vi "Add_DB_info_to_Raw_Data.vi"() -> (0 "Filename":path, 1 "Channel names":string[](array[string]), 2 "Valid File?":bool, 3 "Ch Values":string[][](table))   [LabVIEW 2010]
panel:
  in  "Comment to add":string=" Manually removed"
  in  "Scale Channels":bool
  in  "Scaling Factor":dbl[](array[numeric]) format="%.4f"
  in  "Channel Numbers":i32[](array[numeric])
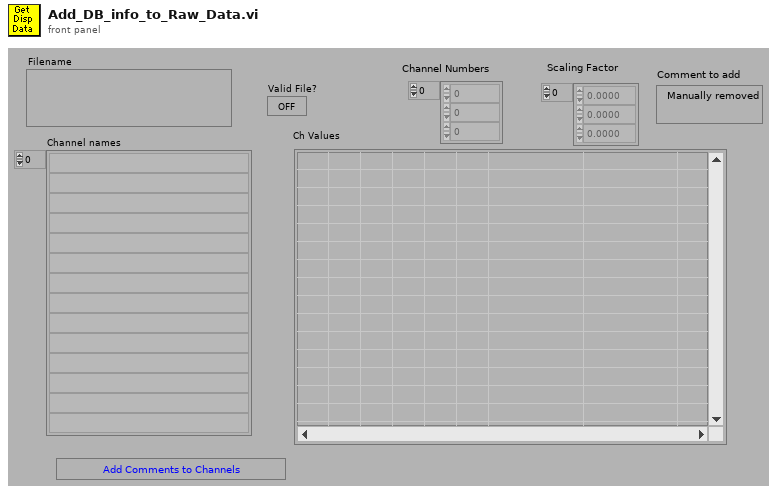
[diagram p1: front panel]
types:
  T1 = enum32{"existing file", "new file", "new or existing file", "existing dir", "new dir", "new or existing dir", "existing file (use LLBs)", "new file (use LLBs)", "new or existing file (use LLBs)", "new or existing file or directory (use LLBs)"}
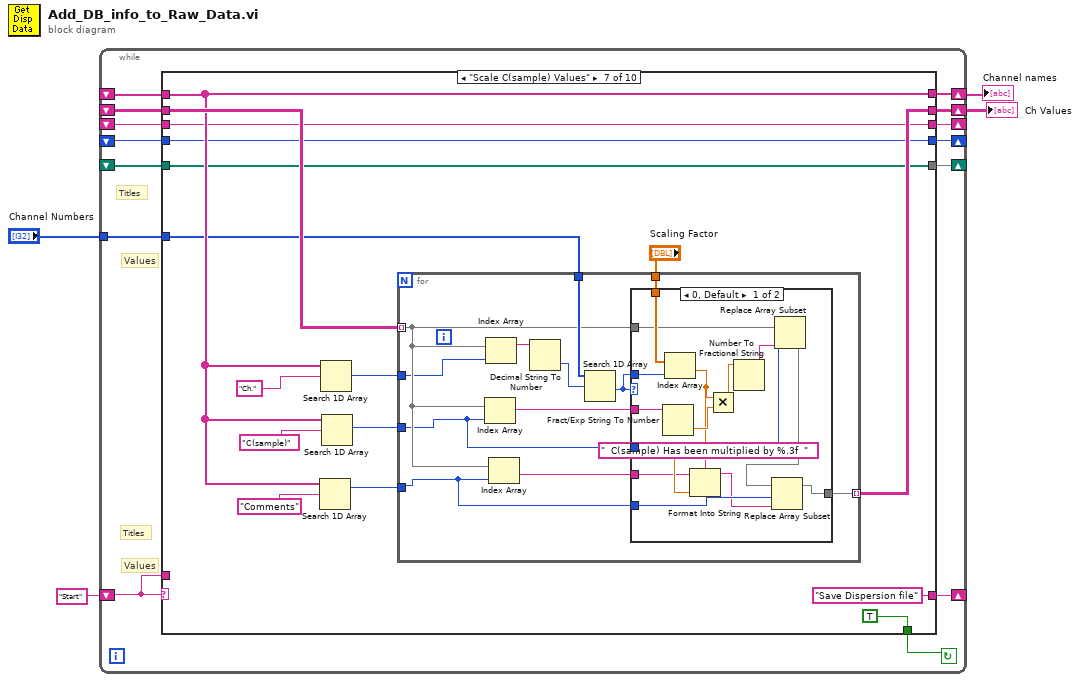
[diagram p0: block diagram]
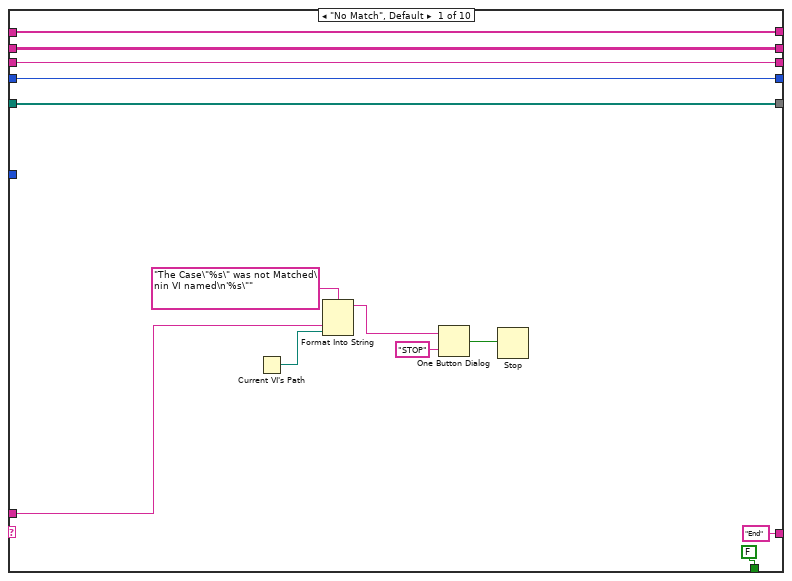
[diagram p2: hidden frame]
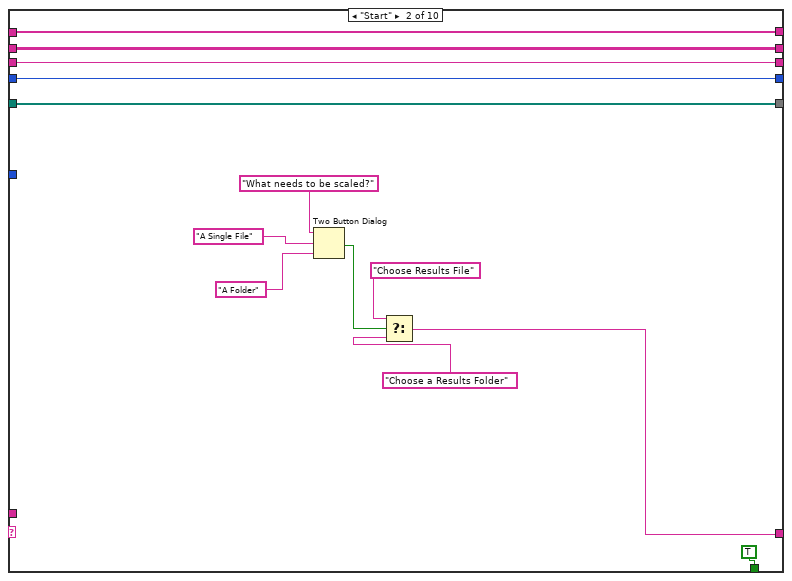
[diagram p3: hidden frame]
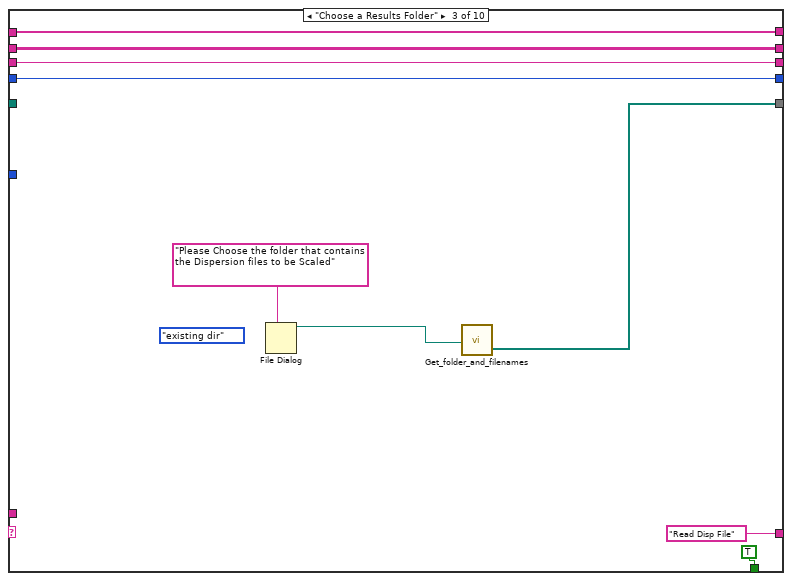
[diagram p4: hidden frame]
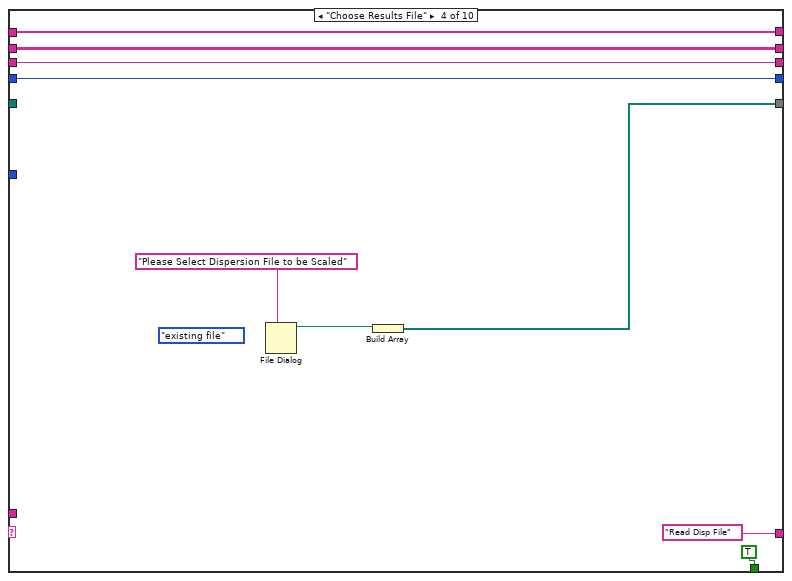
[diagram p5: hidden frame]
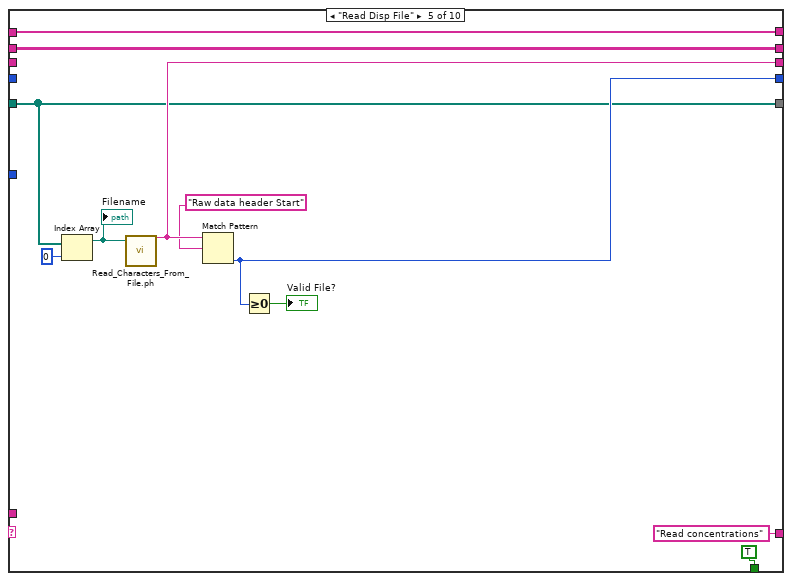
[diagram p6: hidden frame]
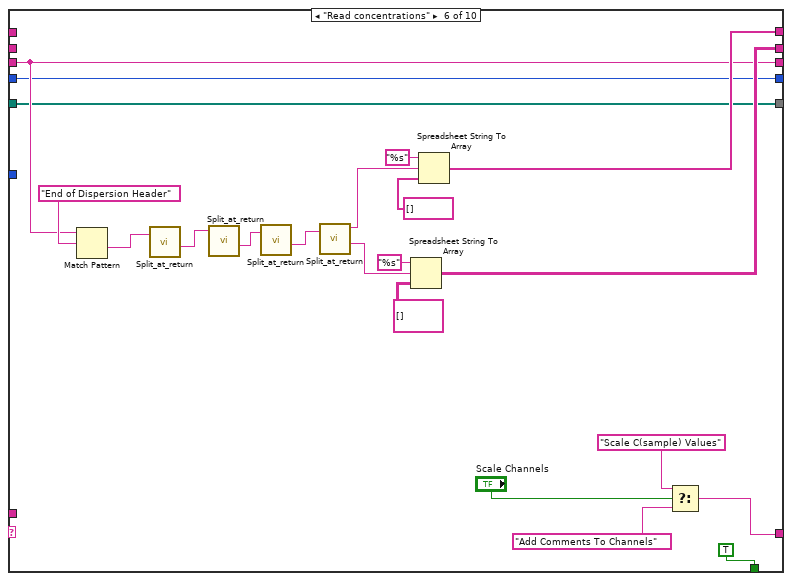
[diagram p7: hidden frame]
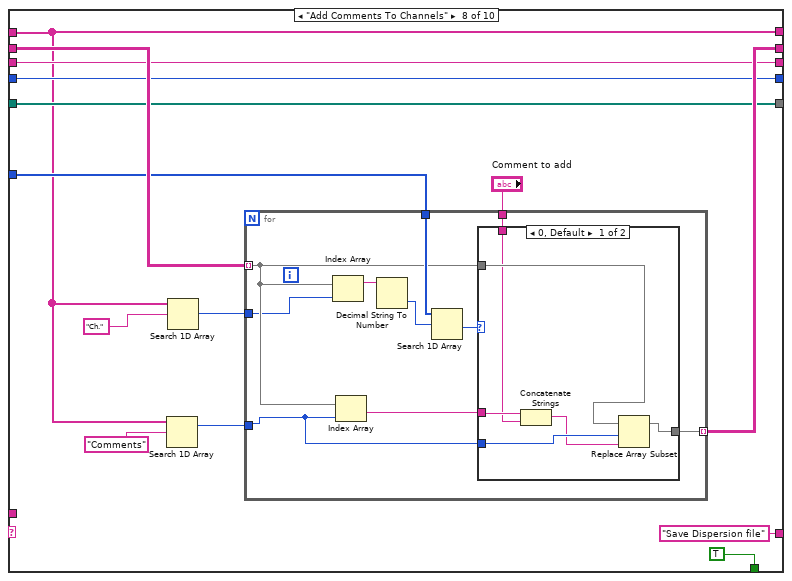
[diagram p9: hidden frame]
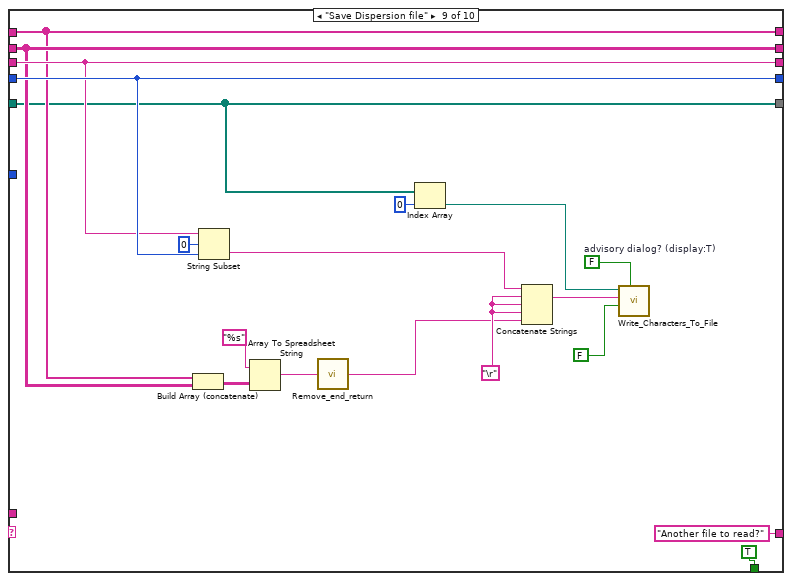
[diagram p11: hidden frame]
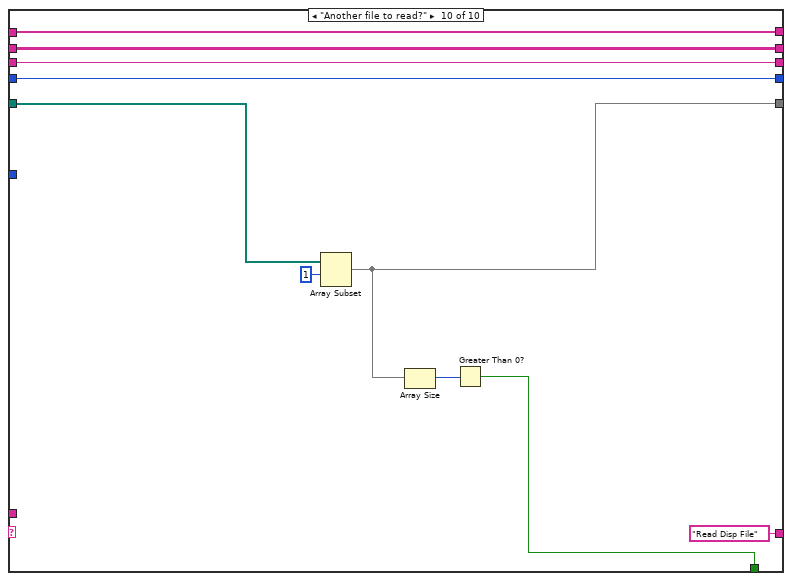
[diagram p12: hidden frame]
diagram:
  n1 = while {
    tunnel: "Channel Numbers" -> [w5]
    shift-left: _ -> [w7]
    shift-right: [w6] -> _
    shift-left: _ -> [w8]
    shift-right: [w10] -> _
    shift-left: _ -> [w13]
    shift-right: [w14] -> _
    shift-left: _ -> [w9]
    shift-right: [w16] -> w2
    shift-left: _ -> [w15]
    shift-right: [w17] -> w3
    shift-left: "Start" -> [w18]
    shift-right: [w12] -> _
    stop <- w11 continue-if-true
    # "Values"
    # "Titles"
    # "Values"
    # "Titles"
    n2 = case shown="\"Scale C(sample) Values\"" w18 {
      tunnel: w18 -> [w26 _ _ _ _ _ _ _ _ _]
      tunnel: [w23 w42 w51 w60 w71 w81 w100 w139 w182 w196] -> w17
      tunnel: [w24 w43 w52 w61 w70 w82 w101 w146 w183 w195] -> w16
      tunnel: w15 -> [w23 w42 w51 w60 w71 _ w100 w139 w182 w196]
      tunnel: [w25 w44 w53 w62 w72 w80 w99 w145 w187 w194] -> w14
      tunnel: w13 -> [w25 w44 w53 w62 _ w80 w99 w145 w187 w194]
      tunnel: ["End" w32 "Read Disp File" "Read Disp File" "Read concentrations" w75 "Save Dispersion file" "Save Dispersion file" "Another file to read?" "Read Disp File"] -> w12
      tunnel: [FALSE TRUE TRUE TRUE TRUE TRUE TRUE TRUE TRUE w198] -> w11
      tunnel: [w20 w40 w49 w58 w67 w79 w97 w143 w188 w193] -> w10
      tunnel: w9 -> [w24 w43 w52 w61 w70 _ w102 w147 w183 w195]
      tunnel: w8 -> [w20 w40 w49 w58 _ w79 w97 w143 w188 w193]
      tunnel: w7 -> [w19 w39 _ _ w65 w78 w96 w142 w172 w192]
      tunnel: [w19 w39 w46 w55 w65 w78 w96 w142 w172 w190] -> w6
      tunnel: w5 -> [_ _ _ _ _ _ w95 w141 _ _]
      frame "No Match", Default {
        n3 = Current VI's Path() -> (path=w27:path)
        n4 = Format Into String(format string="The Case\"%s\" was not Matched\nin VI named\n'%s\"" ("Format String"), w26, w27) -> (resulting string=w30:string)  [unwired: 2 in, 1 out]
        n5 = One Button Dialog(message=w30, button name ("OK")="STOP") -> (true=w28:bool)
        n6 = Stop(stop? (T)=w28) -> ()
      }
      frame "Start" {
        n7 = Two Button Dialog(message="What needs to be scaled?", 1:"A Folder" ("F button name (\"Cancel\")"), 2:"A Single File" ("T button name (\"OK\")")) -> (T button?=w35:bool)
        n8 = Select(t="Choose Results File", s=w35, f="Choose a Results Folder") -> (s? t:f=w32:string)
      }
      frame "Choose a Results Folder" {
        (unwired) T1."existing dir" ("select mode (2)")
        n9 = File Dialog(7:"Please Choose the folder that contains the Dispersion files to be Scaled" ("prompt")) -> (3:w47:path)  [unwired: 6 in, 3 out]
        n10 = call "Get_folder_and_filenames.vi"("file path (dialog if empty)"=w47) -> ("Files"=w46:path[])  [unwired: 1 out]
      }
      frame "Choose Results File" {
        (unwired) T1."existing file" ("select mode (2)")
        n11 = File Dialog(7:"Please Select Dispersion File to be Scaled" ("prompt")) -> (3:w56:path)  [unwired: 6 in, 3 out]
        n12 = Build Array(w56) -> (w55:path[])
      }
      frame "Read Disp File" {
        n13 = Index Array(array=w65, index=0 ("Index")) -> (element=w64:path)
        "Filename" <- w64
        n14 = call "Read_Characters_From_File.ph.vi"("file path (dialog if empty)"=w64) -> ("character string"=w72:string)  [unwired: 5 in, 3 out]
        n15 = Match Pattern(string=w72, regular expression="Raw data header Start") -> (offset past match=w67:i32)  [unwired: 1 in, 3 out]
        n16 = Greater Or Equal To 0?(x=w67) -> (x >= 0?=→"Valid File?":bool)
      }
      frame "Read concentrations" {
        n17 = Match Pattern(string=w80, regular expression="End of Dispersion Header") -> (after substring=w93:string)  [unwired: 1 in, 3 out]
        n18 = call "Split_at_return.vi"("String"=w93) -> ("after substring"=w92:string)  [unwired: 1 in, 3 out]
        n19 = call "Split_at_return.vi"("String"=w92) -> ("after substring"=w91:string)  [unwired: 1 in, 3 out]
        n20 = call "Split_at_return.vi"("String"=w91) -> ("after substring"=w90:string)  [unwired: 1 in, 3 out]
        n21 = call "Split_at_return.vi"("String"=w90) -> ("before substring"=w87:string, "after substring"=w84:string)  [unwired: 1 in, 2 out]
        n22 = Spreadsheet String To Array(format string="%s", spreadsheet string=w84, array type (2D Dbl)=string[][] [] ("Output Array")) -> (array=w82:string[][])  [unwired: 1 in]
        n23 = Spreadsheet String To Array(format string="%s", spreadsheet string=w87, array type (2D Dbl)=string[] [] ("Output Array")) -> (array=w81:string[])  [unwired: 1 in]
        n24 = Select(t="Scale C(sample) Values", s="Scale Channels", f="Add Comments To Channels") -> (s? t:f=w75:string)
      }
      frame "Scale C(sample) Values" {
        n25 = Search 1D Array(1D array=w100, element="Comments") -> (index of element=w104:i32)  [unwired: 1 in]
        n26 = Search 1D Array(1D array=w100, element="Ch.") -> (index of element=w108:i32)  [unwired: 1 in]
        n27 = Search 1D Array(1D array=w100, element="C(sample)") -> (index of element=w105:i32)  [unwired: 1 in]
        n28 = for {
          tunnel: w108 -> [w115]
          tunnel: w95 -> [w120]
          tunnel: w105 -> [w114]
          tunnel: w104 -> [w113]
          tunnel: "Scaling Factor" -> [w118]
          tunnel: w102 -> [w116] mode=indexing
          tunnel: [w111] -> w101 mode=indexing
          n29 = Index Array(array=w116, index=w114) -> (element=w119:string)
          n30 = Index Array(array=w116, index=w115) -> (element=w121:string)
          n31 = Index Array(array=w116, index=w113) -> (element=w112:string)
          n32 = Decimal String To Number(string=w121) -> (number=w122:i32)  [unwired: 2 in, 1 out]
          n33 = Search 1D Array(1D array=w120, element=w122) -> (index of element=w117:i32)  [unwired: 1 in]
          n34 = case shown="0, Default" w117 {
            tunnel: w116 -> [w131 w138]
            tunnel: w119 -> [w137 _]
            tunnel: w118 -> [w136 _]
            tunnel: w117 -> [w135 _]
            tunnel: w114 -> [w130 _]
            tunnel: w113 -> [w126 _]
            tunnel: w112 -> [w127 _]
            tunnel: [w123 w138] -> w111
            frame 0, Default {
              n35 = Fract/Exp String To Number(string=w137) -> (number=w134:dbl)  [unwired: 3 in, 1 out]
              n36 = Index Array(array=w136, index=w135) -> (element=w128:dbl)
              n37 = Format Into String(format string="  C(sample) Has been multiplied by %.3f  " ("Format String"), initial string=w127, w128) -> (resulting string=w125:string)  [unwired: 1 in, 1 out]
              n38 = Multiply(x=w128, y=w134) -> (x*y=w133:dbl)
              n39 = Number To Fractional String(number=w133) -> (F-format string=w132:string)  [unwired: 3 in]
              n40 = Replace Array Subset(array=w131, new element=w132, index=w130) -> (w129:string[])
              n41 = Replace Array Subset(array=w129, new element=w125, index=w126) -> (w123:string[])
            }
            frame -1 {
            }
          }
        }
      }
      frame "Add Comments To Channels" {
        n42 = Search 1D Array(1D array=w139, element="Comments") -> (index of element=w148:i32)  [unwired: 1 in]
        n43 = Search 1D Array(1D array=w139, element="Ch.") -> (index of element=w150:i32)  [unwired: 1 in]
        n44 = for {
          tunnel: w150 -> [w157]
          tunnel: w141 -> [w160]
          tunnel: w148 -> [w156]
          tunnel: "Comment to add" -> [w159]
          tunnel: w147 -> [w158] mode=indexing
          tunnel: [w155] -> w146 mode=indexing
          n45 = Index Array(array=w158, index=w157) -> (element=w161:string)
          n46 = Index Array(array=w158, index=w156) -> (element=w153:string)
          n47 = Decimal String To Number(string=w161) -> (number=w162:i32)  [unwired: 2 in, 1 out]
          n48 = Search 1D Array(1D array=w160, element=w162) -> (index of element=w154:i32)  [unwired: 1 in]
          n49 = case shown="0, Default" w154 {
            tunnel: w158 -> [w166 w169]
            tunnel: w159 -> [w164 _]
            tunnel: w156 -> [w168 _]
            tunnel: w153 -> [w165 _]
            tunnel: [w167 w169] -> w155
            frame 0, Default {
              n50 = Concatenate Strings(w165, w164) -> (w163:string)
              n51 = Replace Array Subset(array=w166, new element=w163, index=w168) -> (w167:string[])
            }
            frame -1 {
            }
          }
        }
      }
      frame "Save Dispersion file" {
        w173 = FALSE  # advisory dialog? (display:T)
        w184 = "\r"
        n52 = Build Array (concatenate)(w182, w183) -> (w181:string[][])
        n53 = String Subset(string=w187, offset (0)=0, length (rest)=w188) -> (substring=w185:string)
        n54 = Array To Spreadsheet String(array=w181, 3:"%s" ("format string")) -> (spreadsheet string=w179:string)  [unwired: 1 in]
        n55 = call "Remove_end_return.vi"("Input string"=w179) -> ("Output string"=w178:string)
        n56 = Index Array(array=w172, index=0 ("Index")) -> (element=w170:path)
        n57 = Concatenate Strings(w185, w184, w184, w184, w178) -> (w177:string)
        n58 = call "Write_Characters_To_File.vi"("file path (dialog if empty)"=w170, "advisory dialog? (display:T)"=w173, "character string"=w177, "append to file? (new file:F)"=FALSE) -> ()  [unwired: 4 in, 1 out]
      }
      frame "Another file to read?" {
        n59 = Array Subset(array=w192, index=1 ("Array Index")) -> (w190:path[])  [unwired: 1 in]
        n60 = Array Size(array=w190) -> (size(s)=w189:i32)
        n61 = Greater Than 0?(x=w189) -> (x > 0?=w198:bool)
      }
    }
  }
  "Channel names" <- w3
  "Ch Values" <- w2
